vi "Error Write Status.vi"(8 "error in":errorcluster, 10 "Error STS":i32, 11 "Chiller in":refnum<class "Chiller.lvclass">) -> (0 "error out":errorcluster, 3 "Chiller out":refnum<class "Chiller.lvclass">)   [LabVIEW 2023, in "Chiller.lvclass"]
uses:
  Chiller.lvclass
  Chiller.lvclass/Chiller.ctl
  Low Level Capabilities/Error/Error.lvclass
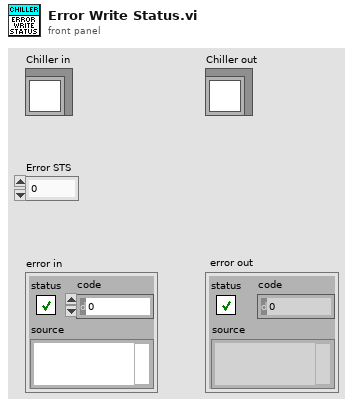
[diagram p1: front panel]
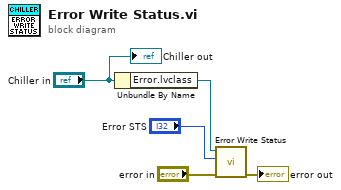
[diagram p0: block diagram]
diagram:
  n1 = Unbundle By Name("Chiller in") -> ("Error.lvclass"=w5:refnum<class "Error.lvclass">)
  n2 = call-dynamic "Error Write Status.vi"("error in"="error in", "Error STS"="Error STS", "Error in"=w5) -> ("error out"=→"error out":errorcluster)  [unwired: 7 in, 1 out]
  "Chiller out" <- "Chiller in"
